vi "Array To Autonomous Commands.vi"(2 "Which":dbl, 3 "Input Array":string[][][](array[string])) -> (0 "Float Output Array":dbl[](array[numeric]), 1 "String Output Array":string[](array[string]))   [LabVIEW 2016]
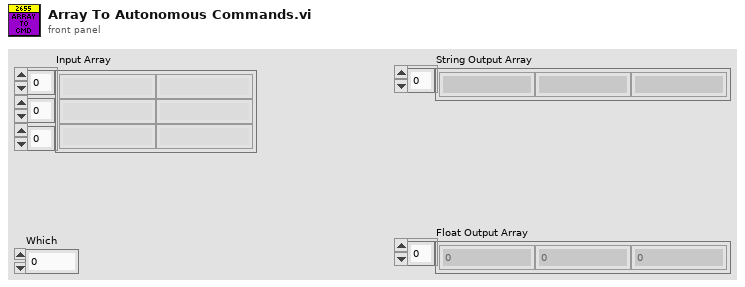
[diagram p1: front panel]
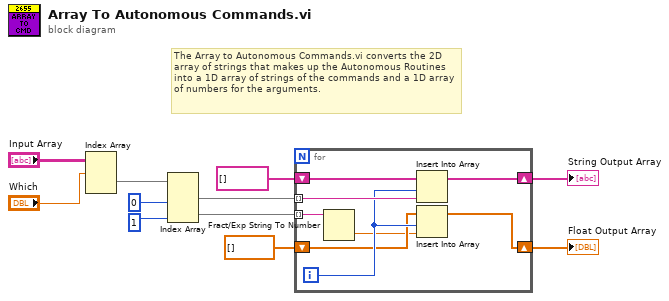
[diagram p0: block diagram]
diagram:
  # "The Array to Autonomous Commands.vi converts the 2D array of strings that makes up the Autonomous Routines into a 1D array of strings of the commands and a 1D array of numbers for the arguments."
  n1 = Index Array(array="Input Array", index (dim 0)="Which") -> (element=w9:string[][])  [unwired: 2 in]
  n2 = Index Array(array=w9, index (col) #1=0, index (col) #2=1) -> (element #1=w6:string[], element #2=w5:string[])  [unwired: 2 in]
  n3 = for {
    tunnel: w6 -> [w19] mode=indexing
    tunnel: w5 -> [w12] mode=indexing
    shift-right: [w17] -> w1
    shift-left: string[] [] ("String Output Array 2") -> [w18]
    shift-right: [w14] -> w2
    shift-left: dbl[] [] ("Float Output Array") -> [w15]
    i -> [w16]
    n4 = Fract/Exp String To Number(string=w12) -> (number=w13:dbl)  [unwired: 3 in, 1 out]
    n5 = Insert Into Array(array=w18, index=w16, new element=w19) -> (w17:string[])
    n6 = Insert Into Array(array=w15, index=w16, new element=w13) -> (w14:dbl[])
  }
  "Float Output Array" <- w2
  "String Output Array" <- w1
